vi "Open 4.vi"(8 "Front Right Motor":T1=enum."Invalid", 9 "Front Left Motor":T1=enum."Invalid", 10 "Rear Right Motor":T1=enum."Invalid", 11 "Rear Left Motor":T1=enum."Invalid") -> (0 "error out":errorcluster, 3 "RobotDriveDevRef":T2={"DevStatus"={"status"=FALSE, "code"=0, "source"=""}, "Motors[]"=[], "Square Inputs"=FALSE, "Max Output"=1.0, "Isochronous"=FALSE})   [LabVIEW 2013]
uses:
  <vilib>/Rock Robotics/SystemInterfaces/DIO/FPGA_DIOPWMChannel.ctl
  <vilib>/Rock Robotics/WPI/RobotDrive/WPI_RobotDriveDevRef.ctl
  <vilib>/Rock Robotics/WPI/MotorControl/WPI_MotorControlDeviceRef.ctl
  <vilib>/Rock Robotics/SystemInterfaces/Typedef/FPGA_TypedefDigitalModule.ctl
  <vilib>/Rock Robotics/WPI/PWM/WPI_PWMDeadband.ctl
  <vilib>/Rock Robotics/WPI/CAN/Jaguar/SubVIs/WPI_CANJaguar_ControlMode.ctl
  <vilib>/Rock Robotics/WPI/PWM/WPI_PWMTransform_ConPane.ctl
  <vilib>/Rock Robotics/WPI/SafetyOutput/WPI_SafetyOutputConfigMenu.ctl
  <vilib>/Rock Robotics/WPI/MotorControl/WPI_MotorControlOpen Jaguar.vi
panel:
  in  "error in (no error)":errorcluster
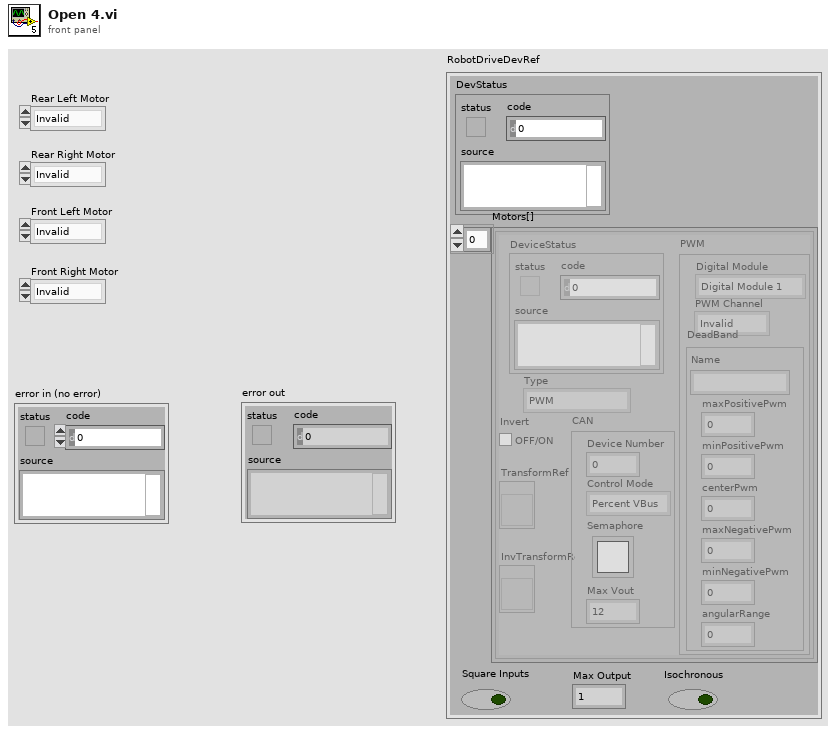
[diagram p1: front panel]
types:
  T1 = typedef "FPGA_DIOPWMChannel.ctl" = enum8{"PWM 1", "PWM 2", "PWM 3", "PWM 4", "PWM 5", "PWM 6", "PWM 7", "PWM 8", "PWM 9", "PWM 10", "Invalid"}
  T2 = typedef "WPI_RobotDriveDevRef.ctl" = cluster{"DevStatus":errorcluster, "Motors[]":T3[], "Square Inputs":bool, "Max Output":dbl, "Isochronous":bool}
  T3 = typedef "WPI_MotorControlDeviceRef.ctl" = cluster{"DeviceStatus":errorcluster, "Type":enum16{"PWM", "CAN"}, "PWM":cluster{"Digital Module":T4, "PWM Channel":T1, "DeadBand":T5}, "CAN":cluster{"Device Number":u8, "Control Mode":T6, "Semaphore":T7, "Max Vout":dbl}, "Invert":bool, "TransformRef":T8, "InvTransformRef":T8}
  T4 = typedef "FPGA_TypedefDigitalModule.ctl" = enum16{"Digital Module 1", "Digital Module 2"}
  T5 = typedef "WPI_PWMDeadband.ctl" = cluster{"Name":string, "maxPositivePwm":i32, "minPositivePwm":i32, "centerPwm":i32, "maxNegativePwm":i32, "minNegativePwm":i32, "angularRange":u16}
  T6 = typedef "WPI_CANJaguar_ControlMode.ctl" = enum8{"Percent VBus", "Current", "Speed", "Position", "Voltage"}
  T7 = typedef "Semaphore RefNum" = refnum<k1>
  T8 = typedef "WPI_PWMTransform_ConPane.ctl" = refnum<vi>
  T9 = typedef "WPI_SafetyOutputConfigMenu.ctl" = enum16{"Enable", "Disable"}
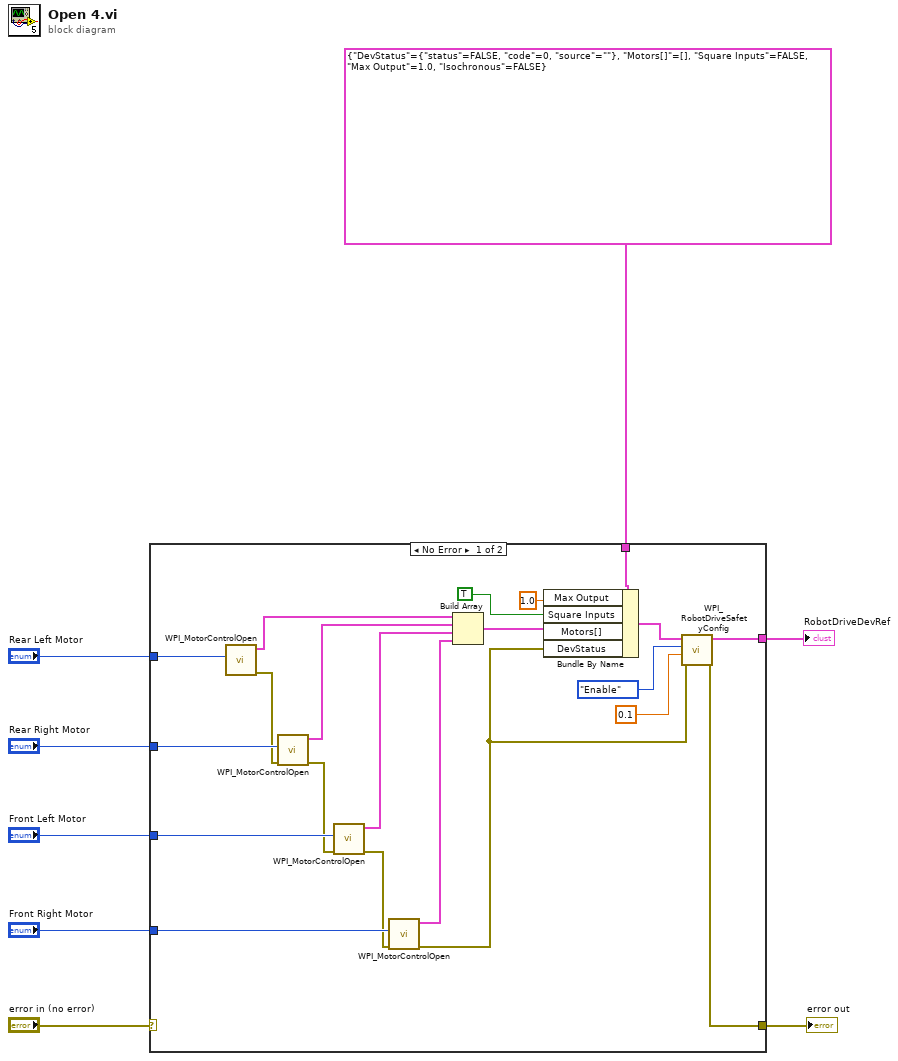
[diagram p0: block diagram]
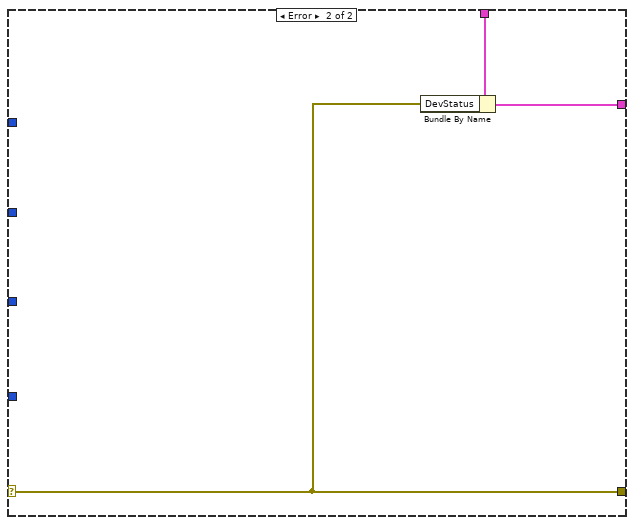
[diagram p2: hidden frame]
diagram:
  n1 = case shown="No Error" "error in (no error)" {
    selector: "error in (no error)" -> [_ w30]
    tunnel: [w11 w31] -> w8
    tunnel: T2 {"DevStatus"={"status"=FALSE, "code"=0, "source"=""}, "Motors[]"=[], "Square Inputs"=FALSE, "Max Output"=1.0, "Isochronous"=FALSE} ("RobotDriveDevRef") -> [w29 w32]
    tunnel: "Rear Left Motor" -> [w27 _]
    tunnel: "Front Right Motor" -> [w24 _]
    tunnel: "Front Left Motor" -> [w25 _]
    tunnel: "Rear Right Motor" -> [w26 _]
    tunnel: [w12 w30] -> w1
    frame No Error {
      n2 = call-poly <vilib>:"WPI_MotorControlOpen.vi"("PWM Channel"=w27) -> ("error out"=w17:errorcluster, "MotorControlDeviceRef"=w23:T3)  [unwired: 6 in, 3 out]
      n3 = call-poly <vilib>:"WPI_MotorControlOpen.vi"("error in (no error)"=w17, "PWM Channel"=w26) -> ("error out"=w18:errorcluster, "MotorControlDeviceRef"=w22:T3)  [unwired: 5 in, 3 out]
      n4 = call-poly <vilib>:"WPI_MotorControlOpen.vi"("error in (no error)"=w18, "PWM Channel"=w25) -> ("error out"=w19:errorcluster, "MotorControlDeviceRef"=w21:T3)  [unwired: 5 in, 3 out]
      n5 = call-poly <vilib>:"WPI_MotorControlOpen.vi"("error in (no error)"=w19, "PWM Channel"=w24) -> ("error out"=w13:errorcluster, "MotorControlDeviceRef"=w20:T3)  [unwired: 5 in, 3 out]
      n6 = Build Array(w23, w22, w21, w20) -> (w16:T3[])
      n7 = Bundle By Name(cluster=w29, "Max Output"=1.0, "Square Inputs"=TRUE ("DestroyPWM?"), "Motors[]"=w16, "DevStatus"=w13) -> (w14:T2)
      n8 = call <vilib>:"WPI_RobotDriveSafetyConfig.vi"("error in (no error)"=w13, "timeout (s)"=0.1, "mode"=WPI_SafetyOutputConfigMenu."Enable", "RobotDriveDevRef"=w14) -> ("error out"=w12:errorcluster, "RobotDriveDevRef"=w11:T2)  [unwired: 6 out]
    }
    frame Error {
      n9 = Bundle By Name(cluster=w32, "DevStatus"=w30) -> (w31:T2)
    }
  }
  "RobotDriveDevRef" <- w8
  "error out" <- w1
